vi "Create and Save Signal.vi"   [LabVIEW 2014]
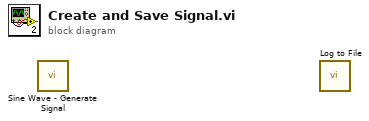
[diagram p0: block diagram]
diagram:
  n1 = call "Sine Wave - Generate Signal.vi"() -> ()  [unwired: 10 in, 2 out]
  n2 = call "Log to File.vi"() -> ()  [unwired: 11 in, 1 out]
